vi "Main.vi"() -> ()   [LabVIEW 2016]
uses:
  Classes/Player/Player.lvclass
  Classes/Match/Match.lvclass/Match.ctl
  Classes/Match/Match.lvclass
panel:
  in  "Play":bool
  in  "Player 2":string
  in  "Player 1":string
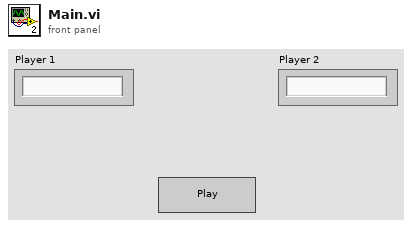
[diagram p1: front panel]
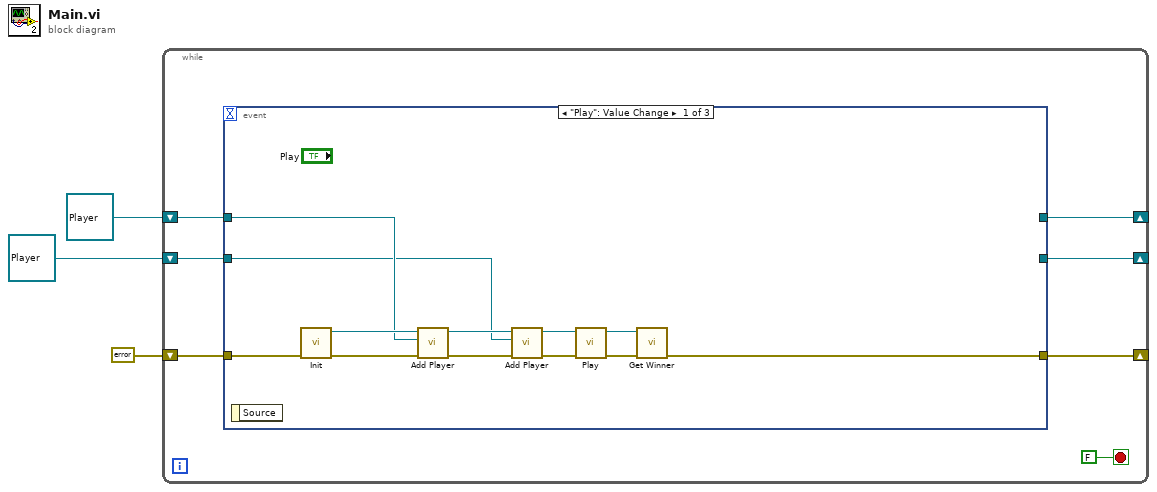
[diagram p0: block diagram]
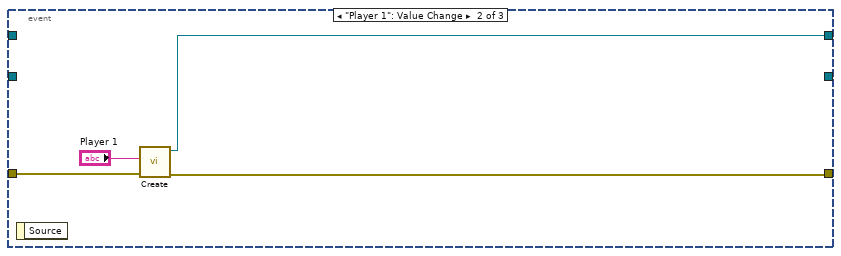
[diagram p2: hidden frame]
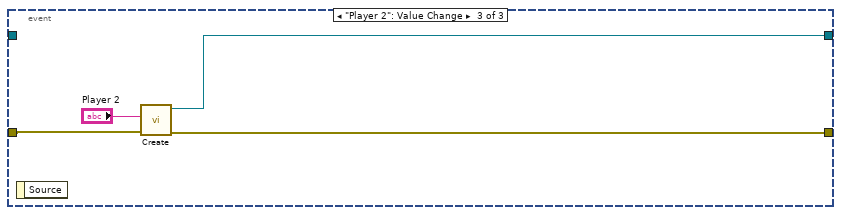
[diagram p3: hidden frame]
diagram:
  n1 = while {
    shift-right: [w8] -> _
    shift-left: errorcluster {"status"=FALSE, "code"=0, "source"=""} ("error out") -> [w9]
    shift-right: [w7] -> _
    shift-left: refnum<class "Player.lvclass"> refnum ("Player.lvclass") -> [w6]
    shift-right: [w5] -> _
    shift-left: refnum<class "Player.lvclass"> refnum ("Player.lvclass") -> [w4]
    stop <- FALSE stop-if-true
    n2 = event shown="[0] \"Play\": Value Change" {
      selector: _ -> [_ _ _]
      dyn-events: _ -> [_ _ _]
      timeout: _ -> [_ _ _]
      tunnel: w9 -> [w19 w26 w30]
      tunnel: [w13 w25 w29] -> w8
      tunnel: [_ w23 _] -> w7
      tunnel: w6 -> [w12 _ _]
      tunnel: [_ _ w28] -> w5
      tunnel: w4 -> [w11 _ _]
      event "Play": Value Change {
        n3 = event-data() -> ()  [unwired: 1 in, 1 out]
        n4 = call "Init.vi"("error in"=w19) -> ("error out"=w18:errorcluster, "Match out"=w20:refnum<class "Match.lvclass">)  [unwired: 9 in]
        n5 = call "Add Player.vi"("error in"=w18, "Player"=w12, "Match in"=w20) -> ("error out"=w21:errorcluster, "Match out"=w22:refnum<class "Match.lvclass">)  [unwired: 7 in]
        n6 = call "Add Player.vi"("error in"=w21, "Player"=w11, "Match in"=w22) -> ("error out"=w16:errorcluster, "Match out"=w17:refnum<class "Match.lvclass">)  [unwired: 7 in]
        n7 = call "Play.vi"("error in (no error)"=w16, "Match in"=w17) -> ("error out"=w15:errorcluster, "Match out"=w14:refnum<class "Match.lvclass">)  [unwired: 8 in]
        n8 = call "Get Winner.vi"("error in (no error)"=w15, "Match in"=w14) -> ("error out"=w13:errorcluster)  [unwired: 7 in, 2 out]
      }
      event "Player 1": Value Change {
        n9 = event-data() -> ()  [unwired: 1 in, 1 out]
        n10 = call "Create.vi"("error in (no error)"=w26, "Player name"="Player 1") -> ("error out"=w25:errorcluster, "Player.lvclass"=w23:refnum<class "Player.lvclass">)  [unwired: 8 in]
      }
      event "Player 2": Value Change {
        n11 = event-data() -> ()  [unwired: 1 in, 1 out]
        n12 = call "Create.vi"("error in (no error)"=w30, "Player name"="Player 2") -> ("error out"=w29:errorcluster, "Player.lvclass"=w28:refnum<class "Player.lvclass">)  [unwired: 8 in]
      }
    }
  }
